vi "PointDistance.vi"(1 "Point 2":cluster{"x":dbl, "y":dbl}, 2 "Point 1":cluster{"x":dbl, "y":dbl}) -> (0 "Distance":dbl)   [LabVIEW 2015, in "Navigation2017.lvlib" / "Navigation2017-util.lvlib"]
doc: "Finds distance between two 2D points."
uses:
  Navigation2017-util.lvlib
panel:
  # "Finds distance between 2 2D points."
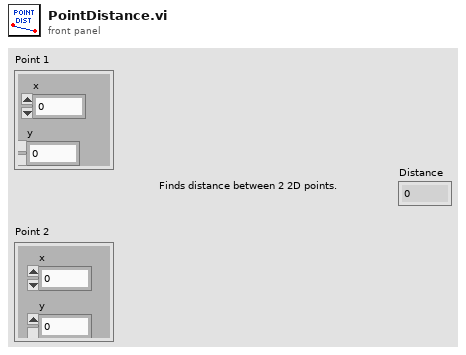
[diagram p1: front panel]
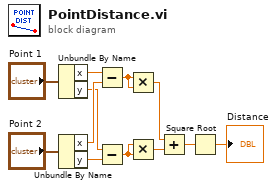
[diagram p0: block diagram]
diagram:
  n1 = Unbundle By Name("Point 1") -> ("x"=w6:dbl, "y"=w3:dbl)
  n2 = Unbundle By Name("Point 2") -> ("x"=w5:dbl, "y"=w2:dbl)
  n3 = Subtract(x=w6, y=w5) -> (x-y=w4:dbl)
  n4 = Subtract(x=w3, y=w2) -> (x-y=w1:dbl)
  n5 = Multiply(x=w4, y=w4) -> (x*y=w12:dbl)
  n6 = Multiply(x=w1, y=w1) -> (x*y=w11:dbl)
  n7 = Add(x=w12, y=w11) -> (x+y=w10:dbl)
  n8 = Square Root(x=w10) -> (sqrt(x)=→"Distance":dbl)
